vi "SaveFileToCSV(subVI).vi"(1 "Typ signálu":string, 2 "Signál":waveform(dbl)) -> (0 "error out":errorcluster)   [LabVIEW 2026]
uses:
  <vilib>/Utility/file.llb/Write Delimited Spreadsheet (DBL).vi
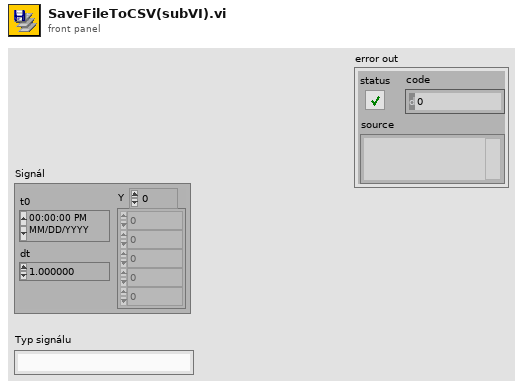
[diagram p1: front panel]
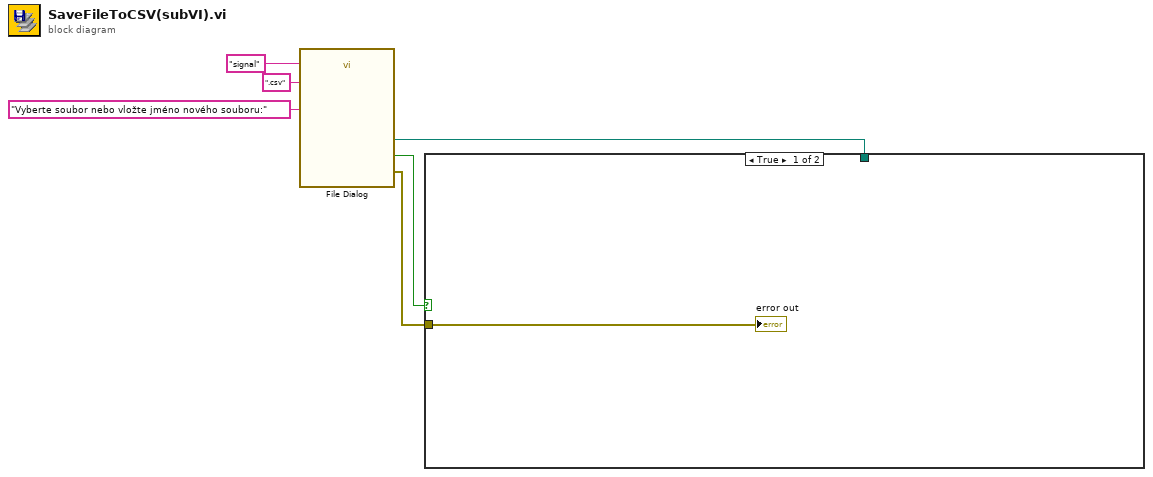
[diagram p0: block diagram]
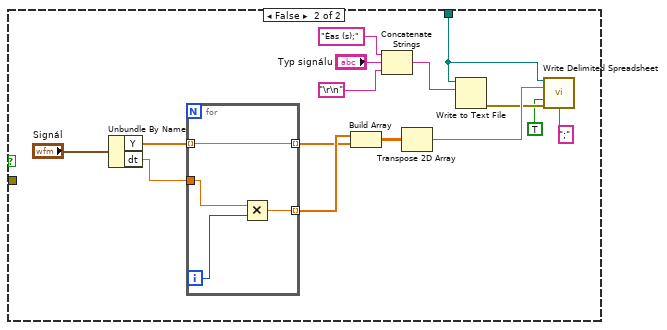
[diagram p2: hidden frame]
diagram:
  n1 = call "File Dialog"("prompt"="Vyberte soubor nebo vložte jméno nového souboru:", "default name"="signal", "pattern (all files)"=".csv") -> ("selected path"=w3:path, "cancelled"=w2:bool, "error out"=w1:errorcluster)  [unwired: 9 in, 1 out]
  n2 = case shown="True" w2 {
    tunnel: w3 -> [_ w8]
    tunnel: w1 -> [w7 _]
    frame True {
      "error out" <- w7
    }
    frame False {
      n3 = Unbundle By Name("Signál") -> ("Y"=w21:dbl[], "dt"=w20:dbl)
      n4 = for {
        tunnel: w21 -> [w26] mode=indexing
        tunnel: w20 -> [w25]
        tunnel: [w26] -> w18 mode=indexing
        tunnel: [w23] -> w19 mode=indexing
        i -> [w24]
        n5 = Multiply(x=w25, y=w24) -> (x*y=w23:dbl)
      }
      n6 = Build Array(w19, w18) -> (w17:dbl[][])
      n7 = Concatenate Strings("Èas (s);" ("string"), "Typ signálu", "\r\n") -> (w11:string)
      n8 = Transpose 2D Array(2D array=w17) -> (transposed array=w13:dbl[][])
      n9 = Write to Text File(file (use dialog)=w8, text=w11) -> (error out=w10:errorcluster)  [unwired: 2 in, 2 out]
      n10 = call-poly <vilib>:"Write Delimited Spreadsheet.vi"("file path (dialog if empty)"=w8, "2D data"=w13, "append to file? (new file:F)"=TRUE, "error in (no error)"=w10, "delimiter (\\t)"=";" ("delimiter (\\t)")) -> ()  [unwired: 9 in, 2 out]
    }
  }
